vi "Read Tektronix WFM impl dimention.vi"(8 "Error In":errorcluster, 10 "offset (in bytes) (0)":i64, 11 "WFM file ref":T1={"refnum"=refnum, "byte order"=enum."little-endian", "Version"=0}) -> (0 "Error Out":errorcluster, 2 "Dimension":T2, 3 "WFM file ref out":T1={"refnum"=refnum, "byte order"=enum."little-endian", "Version"=0})   [LabVIEW 2015]
uses:
  WFM impl dimension.ctl
  WFM file ref.ctl
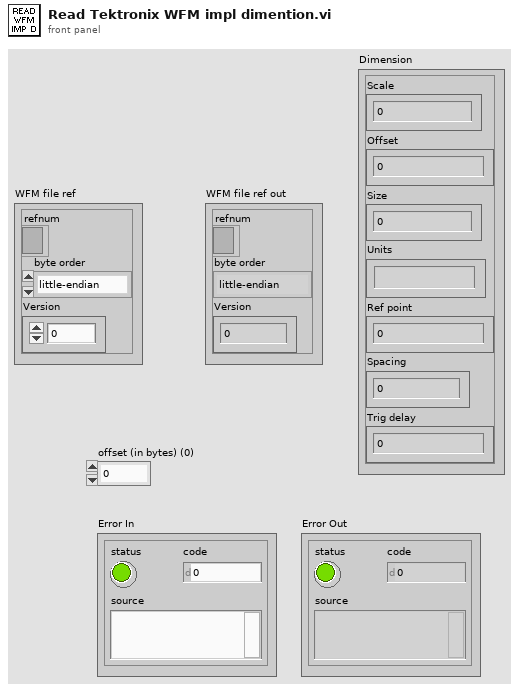
[diagram p1: front panel]
types:
  T1 = typedef "WFM file ref.ctl" = cluster{"refnum":refnum<file>, "byte order":enum16{"big-endian, network order", "native, host order", "little-endian"}, "Version":i32}
  T2 = typedef "WFM impl dimension.ctl" = cluster{"Scale":dbl, "Offset":dbl, "Size":i32, "Units":string, "Ref point":dbl, "Spacing":i32, "Trig delay":dbl}
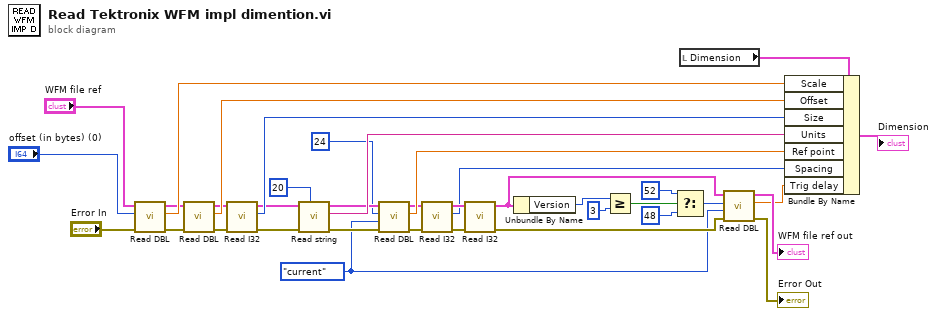
[diagram p0: block diagram]
diagram:
  w1 = enum16{"start", "end", "current"}."current" ("from (0:start)")
  n1 = call "Read DBL.vi"("Error In"="Error In", "offset (in bytes) (0)"="offset (in bytes) (0)", "WFM file ref"="WFM file ref") -> ("Error Out"=w35:errorcluster, "data"=w36:dbl, "WFM file ref out"=w34:T1)  [unwired: 6 in]
  n2 = call "Read DBL.vi"("Error In"=w35, "WFM file ref"=w34) -> ("Error Out"=w31:errorcluster, "data"=w33:dbl, "WFM file ref out"=w32:T1)  [unwired: 7 in]
  n3 = call "Read I32.vi"("Error In"=w31, "WFM file ref"=w32) -> ("Error Out"=w29:errorcluster, "data"=w30:i32, "WFM file ref out"=w28:T1)  [unwired: 7 in]
  n4 = call "Read string.vi"("count (1)"=20, "Error In"=w29, "WFM file ref"=w28) -> ("Error Out"=w23:errorcluster, "data"=w26:string, "WFM file ref out"=w24:T1)  [unwired: 6 in]
  n5 = call "Read DBL.vi"("Error In"=w23, "from (0:start)"=w1, "offset (in bytes) (0)"=i64 24, "WFM file ref"=w24) -> ("Error Out"=w19:errorcluster, "data"=w22:dbl, "WFM file ref out"=w21:T1)  [unwired: 5 in]
  n6 = call "Read I32.vi"("Error In"=w19, "WFM file ref"=w21) -> ("Error Out"=w18:errorcluster, "data"=w17:i32, "WFM file ref out"=w20:T1)  [unwired: 7 in]
  n7 = call "Read I32.vi"("Error In"=w18, "WFM file ref"=w20) -> ("Error Out"=w12:errorcluster, "WFM file ref out"=w9:T1)  [unwired: 7 in, 1 out]
  n8 = Unbundle By Name(w9) -> ("Version"=w8:i32)
  n9 = Greater Or Equal?(x=w8, y=3) -> (x >= y?=w6:bool)
  n10 = Select(t=i64 52, s=w6, f=i64 48) -> (s? t:f=w3:i64)
  n11 = local read "Dimension"() -> (w15:T2)
  n12 = call "Read DBL.vi"("Error In"=w12, "from (0:start)"=w1, "offset (in bytes) (0)"=w3, "WFM file ref"=w9) -> ("Error Out"=→"Error Out":errorcluster, "data"=w10:dbl, "WFM file ref out"=→"WFM file ref out":T1)  [unwired: 5 in]
  n13 = Bundle By Name(cluster=w15, "Scale"=w36, "Offset"=w33, "Size"=w30, "Units"=w26, "Ref point"=w22, "Spacing"=w17, "Trig delay"=w10) -> (→"Dimension":T2)
